vi "Begin.vi"() -> (0 "error out":errorcluster)   [LabVIEW 2013]
doc: "Called before other user functions, this VI is expected to open initial I/O refnums, load in file data, and do all program initialization. Notice that the <B>error out</B> terminal is simply used for data flow. Wiring it to other structures or subVIs ensures that this VI runs first."
uses:
  <vilib>/Rock Robotics/WPI/DriverStation/WPI_DriverStationRobotMode2.ctl
  <vilib>/Rock Robotics/WPI/Joystick/WPI_JoystickDeviceEnum.ctl
  <vilib>/Rock Robotics/SystemInterfaces/DIO/FPGA_DIOChannel.ctl
  <vilib>/Rock Robotics/WPI/Encoder/WPI_EncoderType.ctl
  <vilib>/Rock Robotics/WPI/CAN/Jaguar/SubVIs/WPI_CANJaguar_ControlMode.ctl
  <vilib>/Rock Robotics/WPI/CAN/Jaguar/SubVIs/WPI_CANJaguar_LimitMode.ctl
  <vilib>/Rock Robotics/SystemInterfaces/Typedef/FPGA_TypedefDigitalModule.ctl
  <vilib>/Rock Robotics/SystemInterfaces/DIO/FPGA_DIOPWMChannel.ctl
  Robot Global Data.vi
  <vilib>/Rock Robotics/WPI/RobotDrive/WPI_RobotDriveOpen4MotorWithCANJaguar.vi
  <vilib>/Rock Robotics/WPI/Counter/WPI_CounterDigitalInputToDigitalSource.vi
  <vilib>/Rock Robotics/WPI/MotorControl/WPI_MotorControlOpenCANJaguar.vi
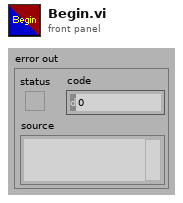
[diagram p1: front panel]
types:
  T1 = typedef "FPGA_DIOPWMChannel.ctl" = enum8{"PWM 1", "PWM 2", "PWM 3", "PWM 4", "PWM 5", "PWM 6", "PWM 7", "PWM 8", "PWM 9", "PWM 10", "Invalid"}
  T2 = typedef "FPGA_TypedefDigitalModule.ctl" = enum16{"Digital Module 1", "Digital Module 2"}
  T3 = typedef "WPI_CANJaguar_LimitMode.ctl" = enum16{"Switch Inputs Only", "Soft Position Limits"}
  T4 = typedef "WPI_CANJaguar_ControlMode.ctl" = enum8{"Percent VBus", "Current", "Speed", "Position", "Voltage"}
  T5 = typedef "WPI_EncoderType.ctl" = enum16{"1x", "2x", "4x"}
  T6 = typedef "FPGA_DIOChannel.ctl" = enum8{"DIO 1", "DIO 2", "DIO 3", "DIO 4", "DIO 5", "DIO 6", "DIO 7", "DIO 8", "DIO 9", "DIO 10", "DIO 11", "DIO 12", "DIO 13", "DIO 14", "Invalid"}
  T7 = typedef "WPI_JoystickDeviceEnum.ctl" = enum16{"USB 1", "USB 2", "USB 3", "USB 4", "Kinect 1", "Kinect 2"}
  T8 = typedef "WPI_DriverStationRobotMode2.ctl" = enum16{"Autonomous Disabled", "Autonomous Enabled", "Teleop Disabled", "Teleop Enabled", "Timeout", "Finish", "Test Disabled", "Test Enabled"}
  T9 = typedef "WPI_JoystickDevRef.ctl" = cluster{"Device":T7}
  T10 = typedef "WPI_RobotDriveDevRef.ctl" = cluster{"DevStatus":errorcluster, "Motors[]":T11[], "Square Inputs":bool, "Max Output":dbl, "Isochronous":bool}
  T11 = typedef "WPI_MotorControlDeviceRef.ctl" = cluster{"DeviceStatus":errorcluster, "Type":enum16{"PWM", "CAN"}, "PWM":cluster{"Digital Module":T2, "PWM Channel":T1, "DeadBand":T12}, "CAN":cluster{"Device Number":u8, "Control Mode":T4, "Semaphore":T13, "Max Vout":dbl}, "Invert":bool, "TransformRef":T14, "InvTransformRef":T14}
  T12 = typedef "WPI_PWMDeadband.ctl" = cluster{"Name":string, "maxPositivePwm":i32, "minPositivePwm":i32, "centerPwm":i32, "maxNegativePwm":i32, "minNegativePwm":i32, "angularRange":u16}
  T13 = typedef "Semaphore RefNum" = refnum<k1>
  T14 = typedef "WPI_PWMTransform_ConPane.ctl" = refnum<vi>
  T15 = typedef "WPI_DigitalInputDevRef.ctl" = cluster{"DevStatus":errorcluster, "DIO Channel":T6, "Digital Module":T2}
  T16 = typedef "FPGA_CounterEncoderSourceConvertionLVSourceType.ctl" = cluster{"DevStatus":errorcluster, "AnalogTriggerMode?":bool, "DigitalMode":cluster{"Digital Module":T2, "DIO Channel":T17}, "AnalogTriggerMode":cluster{"AnalogTriggerIndex":T18, "OutputType":T19}}
  T17 = typedef "FPGA_DIODigitalSourceChannel.ctl" = enum8{"DIO 1", "DIO 2", "DIO 3", "DIO 4", "DIO 5", "DIO 6", "DIO 7", "DIO 8", "DIO 9", "DIO 10", "DIO 11", "DIO 12", "DIO 13", "DIO 14", "Disabled"}
  T18 = typedef "FPGA_AnalogTriggerIndex.ctl" = enum8{"Trig 0", "Trig 1", "Trig 2", "Trig 3", "Trig 4", "Trig 5", "Trig 6", "Trig 7", "Invalid"}
  T19 = typedef "FPGA_AnalogTriggerOutType.ctl" = enum16{"InWindow", "TriggerState", "Rising", "Falling"}
  T20 = typedef "WPI_EncoderDevRef.ctl" = cluster{"DevStatus":errorcluster, "EncoderIndex":T21, "CounterIndex":T22, "DistancePerCount":dbl, "Decoding Type":T5}
  T21 = typedef "FPGA_EncoderIdx.ctl" = enum8{"Enc 0", "Enc 1", "Enc 2", "Enc 3", "Invalid"}
  T22 = typedef "FPGA_CounterCtrSystemIndex.ctl" = enum8{"Ctr 0", "Ctr 1", "Ctr 2", "Ctr 3", "Ctr 4", "Ctr 5", "Ctr 6", "Ctr 7", "Invalid"}
  T23 = typedef "WPI_ServoDeviceRef.ctl" = cluster{"DeviceStatus":errorcluster, "Digital Module":T2, "PWM Channel":T1, "DeadBand":T12}
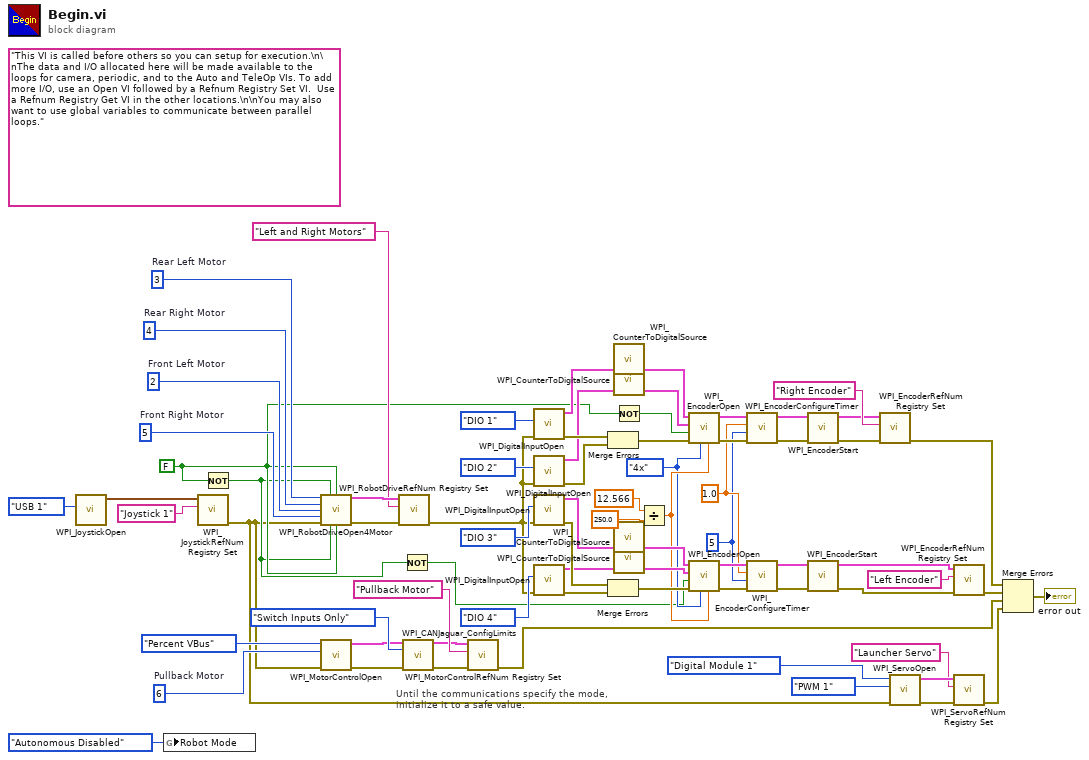
[diagram p0: block diagram]
diagram:
  w15 = u8 6  # Pullback Motor
  w27 = u8 5 ("Number Samples to Average")
  w28 = 1.0 ("Minimum Rate")
  w21 = FALSE ("Rear Left Motor Inverted")
  w37 = u8 5  # Front Right Motor
  w38 = u8 2  # Front Left Motor
  w39 = u8 4  # Rear Right Motor
  w40 = u8 3  # Rear Left Motor
  w41 = WPI_EncoderType."4x" ("Decoding Type")
  (unwired) "This VI is called before others so you can setup for execution.\n\nThe data and I/O allocated here will be made available to the loops for camera, periodic, and to the Auto and TeleOp VIs. To add more I/O, use an Open VI followed by a Refnum Registry Set VI.  Use a Refnum Registry Get VI in the other locations.\n\nYou may also want to use global variables to communicate between parallel loops."
  # "Until the communications specify the mode,\ninitialize it to a safe value."
  n1 = call <vilib>:"WPI_JoystickOpen.vi"("JoystickDevice"=WPI_JoystickDeviceEnum."USB 1") -> ("JoystickDevRef"=w71:T9)  [unwired: 10 in]
  n2 = global write "Robot Global Data.vi" "Robot Mode"(WPI_DriverStationRobotMode2."Autonomous Disabled" ("Robot Mode")) -> ()
  n3 = call <vilib>:"WPI_JoystickRefNum Registry Set.vi"("refnum name"="Joystick 1", "JoystickDevRef"=w71) -> ("error out"=w7:errorcluster)  [unwired: 8 in, 1 out]
  n4 = Not(x=w21) -> (.not. x?=w20:bool)
  n5 = call-poly <vilib>:"WPI_RobotDriveOpen4Motor.vi"("Rear Left Motor"=w40, "Rear Left Motor Inverted"=w20, "Rear Right Motor Inverted"=w21, "Rear Right Motor"=w39, "Front Left Motor"=w38, "Front Right Motor"=w37, "error in (no error)"=w7, "Front Left Motor Inverted"=w20, "Front Right Motor Inverted"=w21) -> ("RobotDriveDevRef"=w68:T10, "error out"=w69:errorcluster)  [unwired: 5 in]
  n6 = call-poly <vilib>:"WPI_MotorControlOpen.vi"("error in (no error)"=w7, "Device Number"=w15, "Control Mode"=WPI_CANJaguar_ControlMode."Percent VBus") -> ("error out"=w16:errorcluster, "MotorControlDeviceRef"=w11:T11)  [unwired: 7 in]
  n7 = call <vilib>:"WPI_RobotDriveRefNum Registry Set.vi"("error in (no error)"=w69, "refnum name"="Left and Right Motors", "RobotDriveDevRef"=w68) -> ("error out"=w26:errorcluster)  [unwired: 7 in, 1 out]
  n8 = Not(x=w20) -> (.not. x?=w19:bool)
  n9 = call <vilib>:"WPI_CANJaguar_ConfigLimits.vi"("CAN Jaguar Ref"=w11, "Limit Mode"=WPI_CANJaguar_LimitMode."Switch Inputs Only", "error in (no error)"=w16) -> ("CAN Jaguar Ref Out"=w9:T11, "error out"=w13:errorcluster)  [unwired: 11 in]
  n10 = call <vilib>:"WPI_MotorControlRefNum Registry Set.vi"("error in (no error)"=w13, "refnum name"="Pullback Motor", "MotorControlDevRef"=w9) -> ("error out"=w8:errorcluster)  [unwired: 7 in, 1 out]
  n11 = call <vilib>:"WPI_DigitalInputOpen.vi"("error in (no error)"=w26, "DIO Channel"=FPGA_DIOChannel."DIO 1") -> ("error out"=w65:errorcluster, "DigitalInputDevRef"=w25:T15)  [unwired: 8 in]
  n12 = call <vilib>:"WPI_DigitalInputOpen.vi"("error in (no error)"=w26, "DIO Channel"=FPGA_DIOChannel."DIO 2") -> ("error out"=w64:errorcluster, "DigitalInputDevRef"=w24:T15)  [unwired: 8 in]
  n13 = call <vilib>:"WPI_DigitalInputOpen.vi"("error in (no error)"=w26, "DIO Channel"=FPGA_DIOChannel."DIO 3") -> ("error out"=w60:errorcluster, "DigitalInputDevRef"=w22:T15)  [unwired: 8 in]
  n14 = call <vilib>:"WPI_DigitalInputOpen.vi"("error in (no error)"=w26, "DIO Channel"=FPGA_DIOChannel."DIO 4") -> ("error out"=w59:errorcluster, "DigitalInputDevRef"=w23:T15)  [unwired: 8 in]
  n15 = Merge Errors(w65, w64) -> (w63:errorcluster)
  n16 = Merge Errors(w60, w59) -> (w58:errorcluster)
  n17 = call-poly <vilib>:"WPI_CounterToDigitalSource.vi"("DigitalInputDevRef"=w25) -> ("Digital Source"=w66:T16)  [unwired: 6 in]
  n18 = call-poly <vilib>:"WPI_CounterToDigitalSource.vi"("DigitalInputDevRef"=w24) -> ("Digital Source"=w62:T16)  [unwired: 6 in]
  n19 = Not(x=w21) -> (.not. x?=w18:bool)
  n20 = call-poly <vilib>:"WPI_CounterToDigitalSource.vi"("DigitalInputDevRef"=w22) -> ("Digital Source"=w61:T16)  [unwired: 6 in]
  n21 = call-poly <vilib>:"WPI_CounterToDigitalSource.vi"("DigitalInputDevRef"=w23) -> ("Digital Source"=w57:T16)  [unwired: 6 in]
  n22 = Divide(x=12.566, y=250.0) -> (x/y=w46:dbl)
  n23 = call <vilib>:"WPI_EncoderOpen.vi"("DistancePerCount"=w46, "Decoding Type"=w41, "error in (no error)"=w63, "Invert Direction (False)"=w18, "BSource"=w62, "ASource"=w66) -> ("error out"=w29:errorcluster, "EncoderDevRef"=w32:T20)  [unwired: 4 in]
  n24 = call <vilib>:"WPI_EncoderOpen.vi"("DistancePerCount"=w46, "Decoding Type"=w41, "error in (no error)"=w58, "Invert Direction (False)"=w19, "BSource"=w57, "ASource"=w61) -> ("error out"=w35:errorcluster, "EncoderDevRef"=w36:T20)  [unwired: 4 in]
  n25 = call <vilib>:"WPI_EncoderConfigureTimer.vi"("error in (no error)"=w29, "Number Samples to Average"=w27, "Minimum Rate"=w28, "EncoderDevRef"=w32) -> ("error out"=w30:errorcluster, "EncoderDevRef"=w31:T20)  [unwired: 6 in]
  n26 = call <vilib>:"WPI_EncoderConfigureTimer.vi"("error in (no error)"=w35, "Number Samples to Average"=w27, "Minimum Rate"=w28, "EncoderDevRef"=w36) -> ("error out"=w33:errorcluster, "EncoderDevRef"=w34:T20)  [unwired: 6 in]
  n27 = call <vilib>:"WPI_EncoderStart.vi"("error in (no error)"=w30, "EncoderDevRef"=w31) -> ("error out"=w42:errorcluster, "EncoderDevRef"=w43:T20)  [unwired: 8 in]
  n28 = call <vilib>:"WPI_EncoderStart.vi"("error in (no error)"=w33, "EncoderDevRef"=w34) -> ("error out"=w44:errorcluster, "EncoderDevRef"=w45:T20)  [unwired: 8 in]
  n29 = call <vilib>:"WPI_EncoderRefNum Registry Set.vi"("error in (no error)"=w42, "refnum name"="Right Encoder", "EncoderDevRef"=w43) -> ("error out"=w56:errorcluster)  [unwired: 7 in, 1 out]
  n30 = call <vilib>:"WPI_ServoOpen.vi"("error in (no error)"=w7, "PWM Channel"=FPGA_DIOPWMChannel."PWM 1", "Digital Module (Module 1)"=FPGA_TypedefDigitalModule."Digital Module 1") -> ("error out"=w4:errorcluster, "ServoDeviceRef"=w3:T23)  [unwired: 7 in]
  n31 = call <vilib>:"WPI_EncoderRefNum Registry Set.vi"("error in (no error)"=w44, "refnum name"="Left Encoder", "EncoderDevRef"=w45) -> ("error out"=w55:errorcluster)  [unwired: 7 in, 1 out]
  n32 = call <vilib>:"WPI_ServoRefNum Registry Set.vi"("error in (no error)"=w4, "refnum name"="Launcher Servo", "ServoDeviceRef"=w3) -> ("error out"=w1:errorcluster)  [unwired: 7 in, 1 out]
  n33 = Merge Errors(w56, w55, w8, w1) -> (→"error out":errorcluster)
